vi "Gyro PID Back Dis.vi"(6 "Target angle":sgl, 7 "Threshold to stop":i32=1200, 8 "Threshold to slow":i32=1000, 9 "Min. speed":i32=20, 10 "Max. speed":i32=40, 11 "EV3 in":T1) -> (3 "EV3 out":T1)   [LabVIEW 2016]
uses:
  <vilib>/NXT/Subs/LVHSConnector.ctl
  <vilib>/NXT/LegoClasses/BrickReference/BrickReference.lvclass
  <vilib>/NXT/Block Support/NXT_OutputPort.ctl
  <vilib>/NXT/NXTIO Xnodes/NXTIONodeSubVIs/LEGOResetMotors.vi
  <vilib>/NXT/Dual Mode Library/Motors/Rotation.vi
  <vilib>/NXT/NXTIO Xnodes/NXTIONodeSubVIs/NXTMotorSteeringOn.vi
  <vilib>/NXT/NXTIO Xnodes/NXTIONodeSubVIs/NXTStopMotors.vi
  <vilib>/NXT/Dual Mode Library/Waits/Wait_Num.vi
  <vilib>/NXT/NXTIO Xnodes/NXTIOXNode/NXTIO.xnode
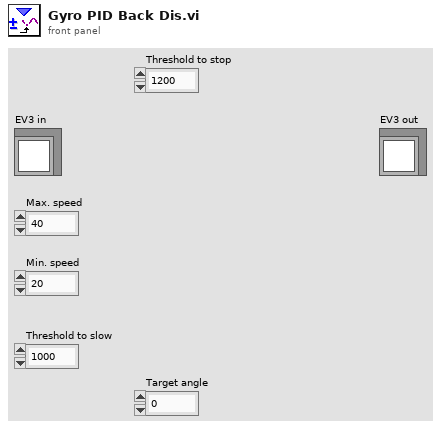
[diagram p1: front panel]
types:
  T1 = typedef "LVHSConnector.ctl" = refnum<class "BrickReference.lvclass">
  T2 = typedef "NXT_OutputPort.ctl" = u8
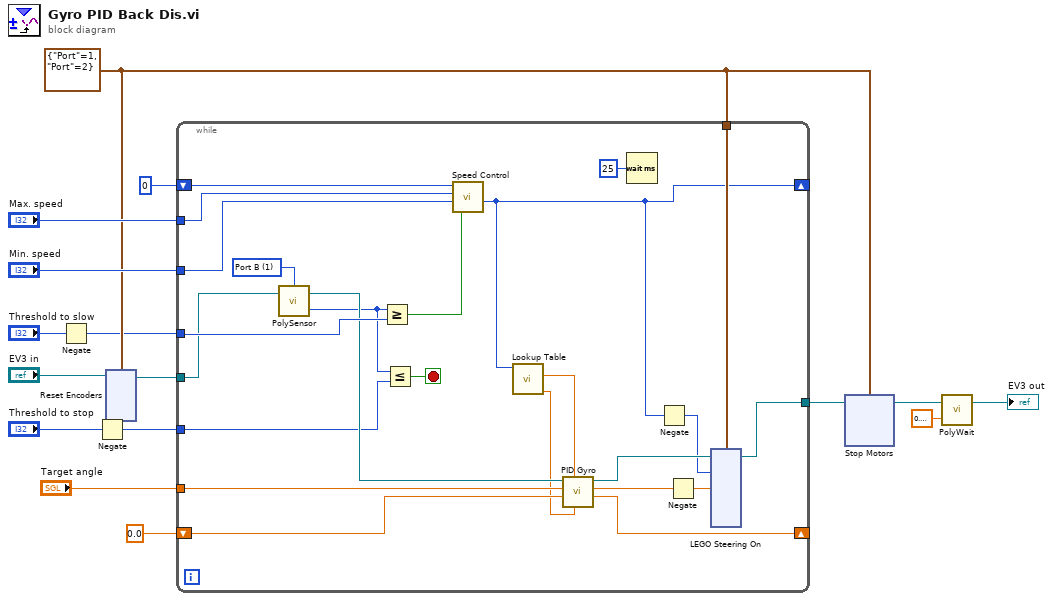
[diagram p0: block diagram]
diagram:
  w6 = cluster{"Port":T2, "Port":T2} {"Port"=1, "Port"=2} ("Motor")
  n1 = Negate(x="Threshold to slow") -> (-x=w2:i32)
  n2 = Negate(x="Threshold to stop") -> (-x=w1:i32)
  n3 = xnode "Reset Encoders"("Motors"=w6, "NXT/EV3"="EV3 in") -> ("NXT/EV3"=w12:T1)
  n4 = while {
    tunnel: w12 -> [w29]
    shift-right: [w40] -> _
    shift-left: sgl 0.0 -> [w23]
    tunnel: "Target angle" -> [w39]
    tunnel: [w36] -> w8
    tunnel: w6 -> [w38]
    shift-right: [w19] -> _
    shift-left: 0 -> [w33]
    tunnel: "Min. speed" -> [w30]
    tunnel: "Max. speed" -> [w32]
    tunnel: w2 -> [w31]
    tunnel: w1 -> [w22]
    stop <- w26 stop-if-true
    w37 = T2 1 items=["Port A", "Port B", "Port C", "Port D"] ("Port (Port A)")
    n5 = call-poly <vilib>:"PolySensor.vi"("NXT/EV3"=w29, "Port (Port A)"=w37) -> ("Angle of Rotation"=w25:i32, "NXT/EV3"=w28:T1)  [unwired: 1 in]
    n6 = Greater Or Equal?(x=w25, y=w31) -> (x >= y?=w27:bool)
    n7 = Less Or Equal?(x=w25, y=w22) -> (x <= y?=w26:bool)
    n8 = call "Speed Control.vi"("Speed Up or Down?"=w27, "Min. speed"=w30, "Max. speed"=w32, "Ini. speed"=w33) -> ("Speed out"=w19:i32)  [unwired: 7 in]
    n9 = call "Lookup Table.vi"("Speed"=w19) -> ("I"=w17:dbl, "P"=w18:dbl)  [unwired: 9 in]
    n10 = call "PID Gyro.vi"("K_i"=w17, "K_p"=w18, "Previous integral"=w23, "Target angle"=w39, "EV3 in"=w28) -> ("New integral"=w40:sgl, "Total error"=w34:sgl, "EV3 out"=w24:T1)  [unwired: 4 in]
    n11 = Wait (ms)(milliseconds to wait=u32 25) -> ()  [unwired: 1 out]
    n12 = Negate(x=w19) -> (-x=w21:i32)
    n13 = Negate(x=w34) -> (-x=w20:sgl)
    n14 = xnode "LEGO Steering On"("Steering 1"=w20, "Power 1"=w21, "Motors"=w38, "NXT/EV3"=w24) -> ("NXT/EV3"=w36:T1)
  }
  n15 = xnode "Stop Motors"("Motors"=w6, "NXT/EV3"=w8) -> ("NXT/EV3"=w7:T1)
  n16 = call-poly <vilib>:"PolyWait.vi"("Time (1 sec)"=sgl 0.2, "NXT/EV3"=w7) -> ("NXT/EV3"=→"EV3 out":T1)  [unwired: 2 in]
